vi "(SubVI) SaveGlimpseHeader.vi"(9 "Header file data 2":T1 {"Pixel depth" items=["8 bits", "16 bits", "Float", "Complex", "RGB", "HSL"]; "time of 1st frame, \nsec since 1/1/04" format="%.2f"}, 10 "Header file data":T1 {"Pixel depth" items=["8 bits", "16 bits", "Float", "Complex", "RGB", "HSL"]; "time of 1st frame, \nsec since 1/1/04" format="%.2f"}, 11 "Select a Folder":path) -> ()   [LabVIEW 2014]
uses:
  4.Other/header ctl/Header file data.ctl
  4.Other/header ctl/Offset table.ctl
  4.Other/header ctl/Offset.ctl
  4.Other/header ctl/file number.ctl
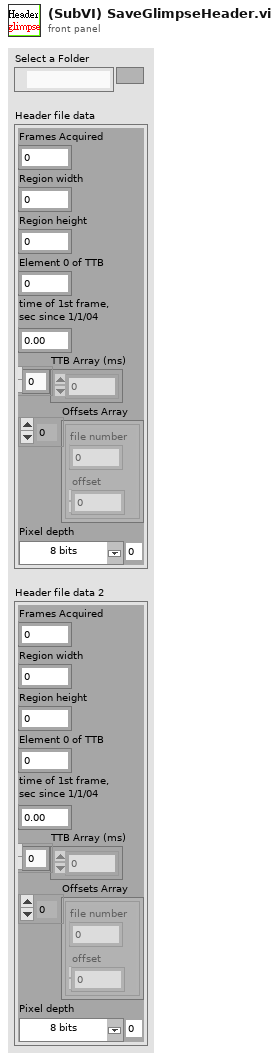
[diagram p1: front panel]
types:
  T1 = typedef "Header file data.ctl" = cluster{"Frames Acquired":u32, "Region width":i32, "Region height":i32, "Element 0 of TTB":u32, "time of 1st frame, \nsec since 1/1/04":dbl, "TTB Array (ms)":u32[], "Offsets Array":T2, "Pixel depth":u32}
  T2 = typedef "Offset table.ctl" = cluster{"offset":T3, "file number":T4}[]
  T3 = typedef "Offset.ctl" = i32
  T4 = typedef "file number.ctl" = u8
  T5 = enum16{"open", "replace", "create", "open or create", "replace or create", "replace or create with confirmation"}
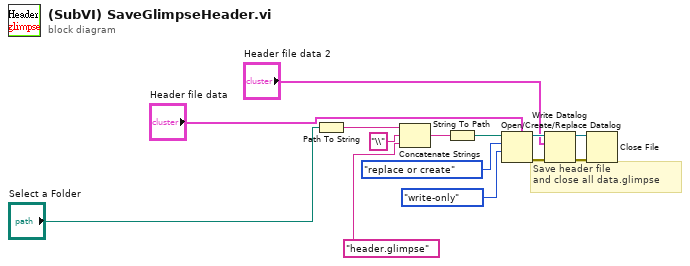
[diagram p0: block diagram]
diagram:
  # "Save header file\nand close all data.glimpse"
  n1 = Path To String(path="Select a Folder") -> (string=w8:string)
  n2 = Concatenate Strings(w8, "\\" ("string"), "header.glimpse" ("string")) -> (w9:string)
  n3 = String To Path(string=w9) -> (path=w11:path)
  n4 = Open/Create/Replace Datalog(5:"Header file data", 9:enum16{"read/write", "read-only", "write-only"}."write-only" ("access (0:read/write)"), 10:T5."replace or create" ("operation (0:open)"), 11:w11) -> (0:w3:errorcluster, 3:w5:refnum<k1>)  [unwired: 1 in, 2 out]
  n5 = Write Datalog(4:w3, 6:"Header file data 2", 7:w5) -> (0:w2:errorcluster, 3:w4:refnum<k1>)
  n6 = Close File(refnum=w4, error in=w2) -> ()  [unwired: 2 out]
